vi "StateSpaceUtil_IsStabilizable.vi"(9 "B":T1, 11 "A":T1) -> (0 "Error":errorcluster, 3 "IsStabilizable":bool, 4 "Eigenvalues":cdb[](array[numeric]), 6 "R rank":i32[](array[numeric]))   [LabVIEW 2019, in "Trajectory_Library.lvlib"]
doc: "Returns true if (A, B) is a stabilizable pair.\n \n(A,B) is stabilizable if and only if the uncontrollable eigenvalues of A, if any, have absolute values less than one, where an eigenvalue is uncontrollable if rank(Lambda - A, B) < n where n is number of states.\n \nInputs:\n - A -- System matrix.\n - B -- nput matrix.\n\nOutputs:\n - IsStablizable -- If the system is stabilizable."
uses:
  Trajectory_Library.lvlib
  <vilib>/Analysis/Matrix/Datatypes/RealMatrix.ctl
  <vilib>/Analysis/Matrix/NI_Matrix.lvlib
panel:
  # "<States, States>"
  # "<States, Inputs>"
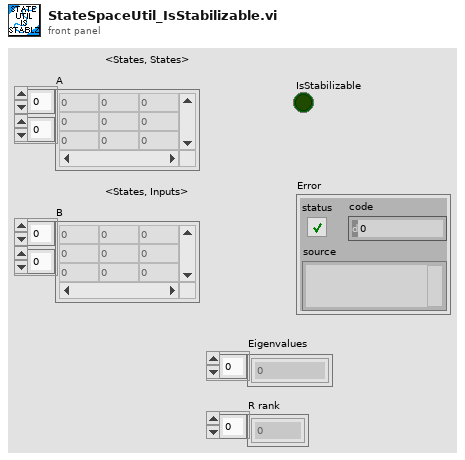
[diagram p1: front panel]
types:
  T1 = typedef "NI_Matrix.lvlib/RealMatrix.ctl" = dbl[][]
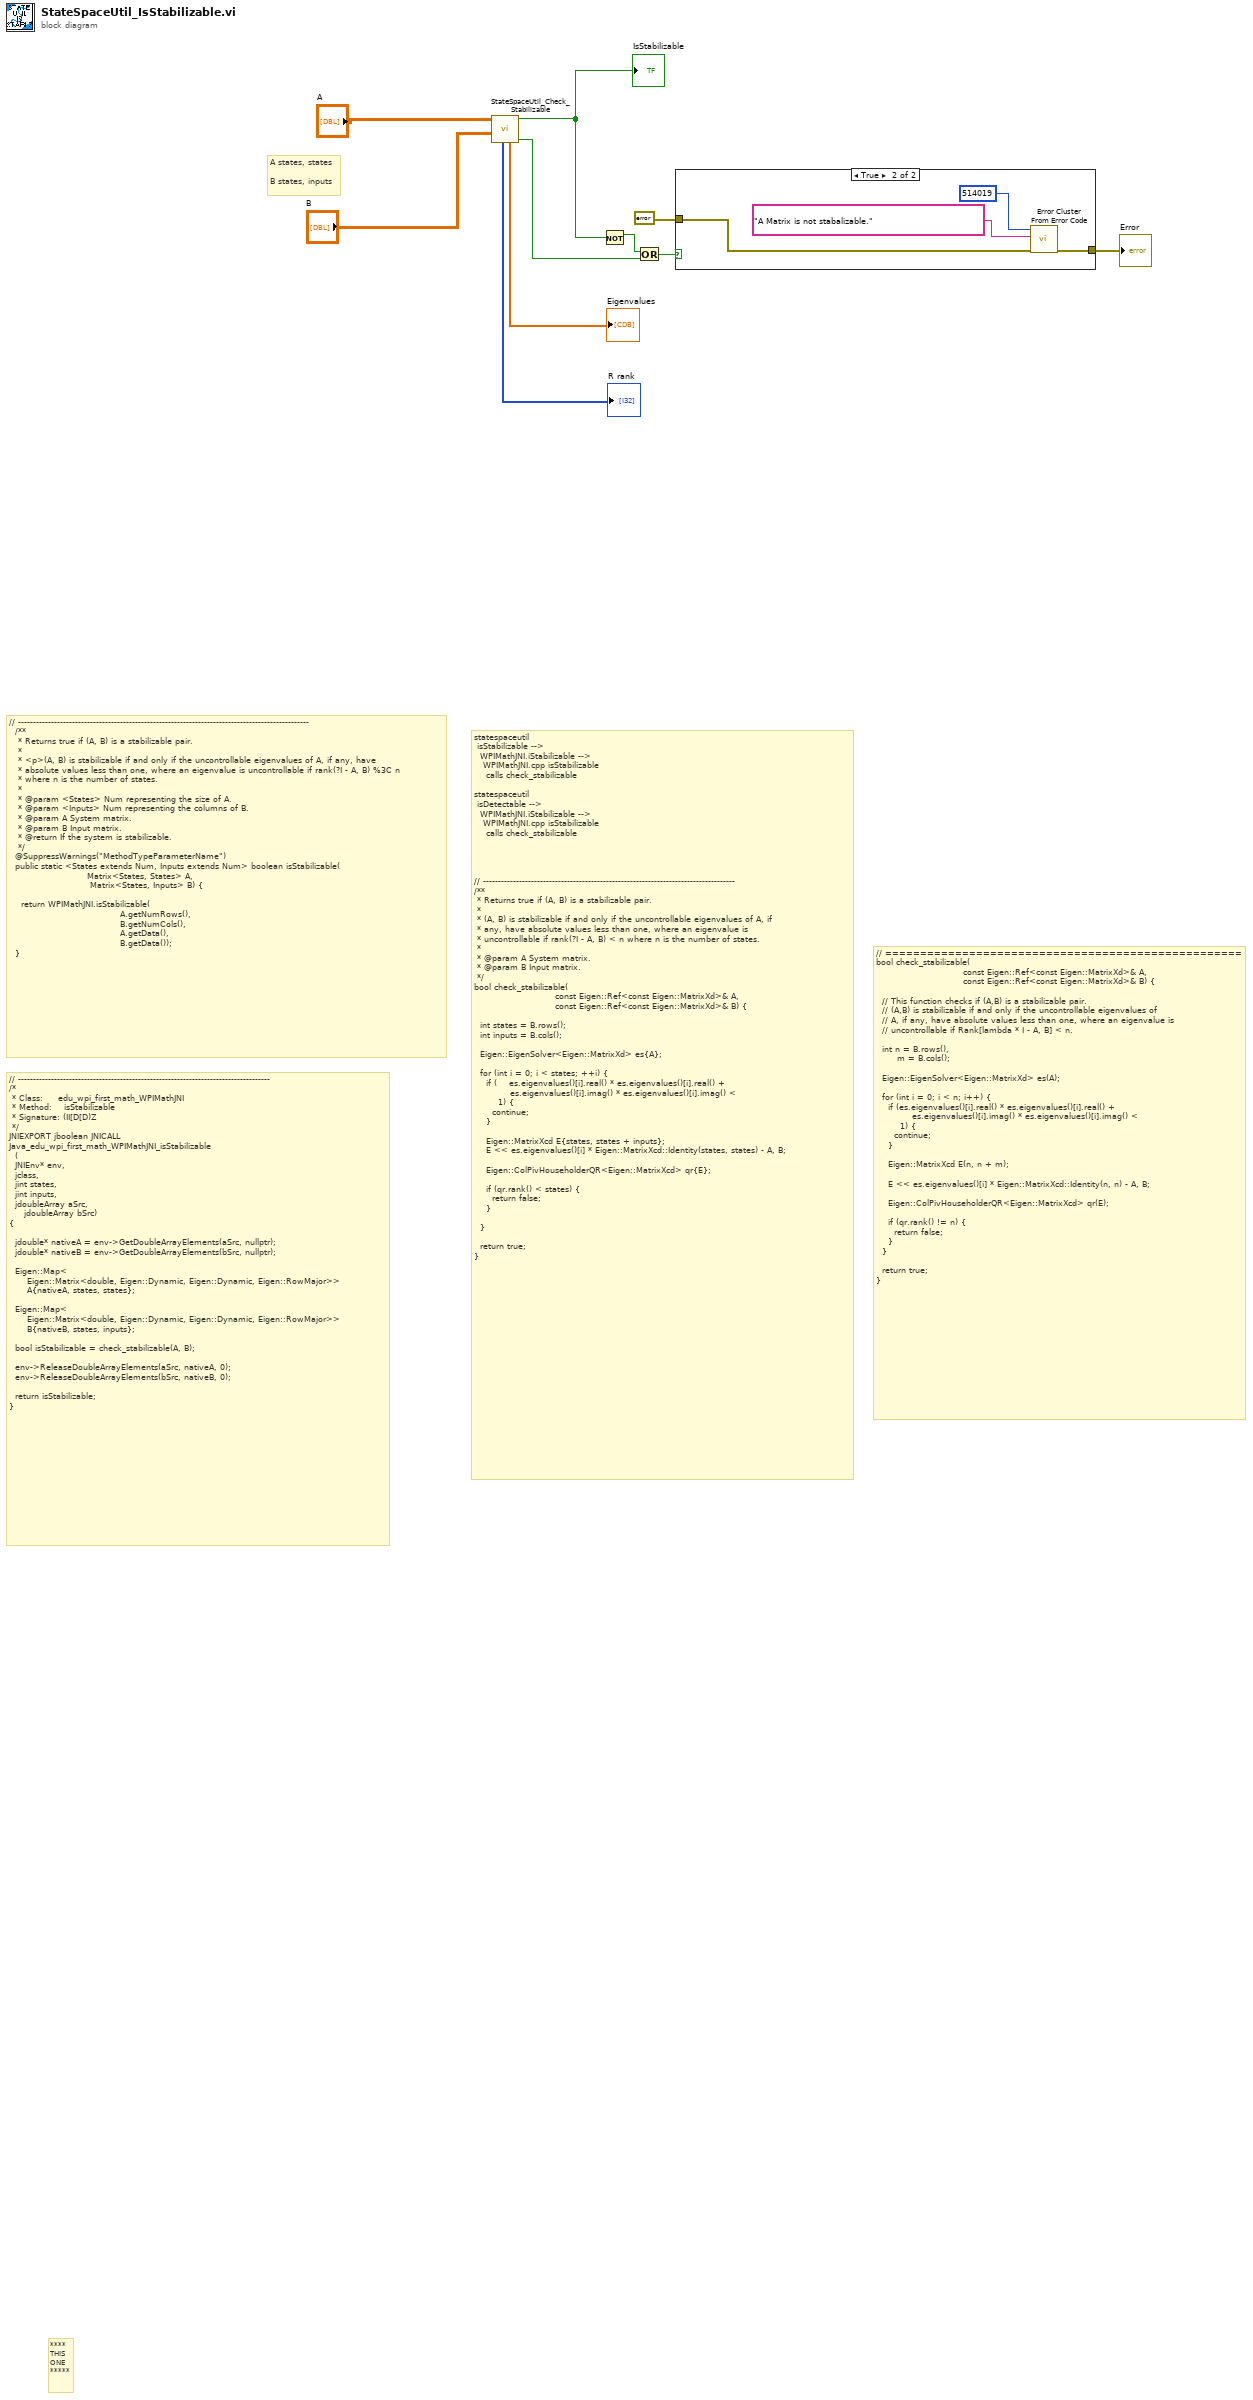
[diagram p0: block diagram]
diagram:
  # "A states, states\n\nB states, inputs"
  # "// ------------------------------------------------------------------------------------\n/*\n * Class:     edu_wpi_first_math_WPIMathJNI\n * Method:    isStabilizable\n * Signature: (II[D[D)Z\n */\nJNIEXPORT jboolean JNICALL\nJava_edu_wpi_first_math_WPIMathJNI_isStabilizable\n  (\n\t\tJNIEnv* env, \n\t\tjclass, \n\t\tjint states, \n\t\tjint inputs, \n\t\tjdoubleArray aSrc,\n   \t\tjdoubleArray bSrc)\n{\n\n  jdouble* nativeA = env->GetDoubleArrayElements(aSrc, nullptr);\n  jdouble* nativeB = env->GetDoubleArrayElements(bSrc, nullptr);\n\n  Eigen::Map<\n      Eigen::Matrix<double, Eigen::Dynamic, Eigen::Dynamic, Eigen::RowMajor>>\n      A{nativeA, states, states};\n\n  Eigen::Map<\n      Eigen::Matrix<double, Eigen::Dynamic, Eigen::Dynamic, Eigen::RowMajor>>\n      B{nativeB, states, inputs};\n\n  bool isStabilizable = check_stabilizable(A, B);\n\n  env->ReleaseDoubleArrayElements(aSrc, nativeA, 0);\n  env->ReleaseDoubleArrayElements(bSrc, nativeB, 0);\n\n  return isStabilizable;\n}"
  # "statespaceutil\n\tisStabilizable --> \n\t\tWPIMathJNI.iStabilizable --> \n\t\t\tWPIMathJNI.cpp isStabilizable  \n\t\t\t\tcalls check_stabilizable\n\nstatespaceutil\n\tisDetectable -->  \n\t\tWPIMathJNI.iStabilizable --> \n\t\t\tWPIMathJNI.cpp isStabilizable\n\t\t\t\tcalls check_stabilizable\n\n\n\n\n// ------------------------------------------------------------------------------------\n/**\n * Returns true if (A, B) is a stabilizable pair.\n *\n * (A, B) is stabilizable if and only if the uncontrollable eigenvalues of A, if\n * any, have absolute values less than one, where an eigenvalue is\n * uncontrollable if rank(?I - A, B) < n where n is the number of states.\n *\n * @param A System matrix.\n * @param B Input matrix.\n */\nbool check_stabilizable(\n                           const Eigen::Ref<const Eigen::MatrixXd>& A,\n                           const Eigen::Ref<const Eigen::MatrixXd>& B) {\n\n  int states = B.rows();\n  int inputs = B.cols();\n\n  Eigen::EigenSolver<Eigen::MatrixXd> es{A};\n\n  for (int i = 0; i < states; ++i) {\n    if (    es.eigenvalues()[i].real() * es.eigenvalues()[i].real() +\n            es.eigenvalues()[i].imag() * es.eigenvalues()[i].imag() <\n        1) {\n      continue;\n    }\n\n    Eigen::MatrixXcd E{states, states + inputs};\n    E << es.eigenvalues()[i] * Eigen::MatrixXcd::Identity(states, states) - A, B;\n\n    Eigen::ColPivHouseholderQR<Eigen::MatrixXcd> qr{E};\n\n    if (qr.rank() < states) {\n      return false;\n    }\n\n  }\n\n  return true;\n}"
  # "// ===================================================\nbool check_stabilizable(\n                             const Eigen::Ref<const Eigen::MatrixXd>& A,\n                             const Eigen::Ref<const Eigen::MatrixXd>& B) {\n\n  // This function checks if (A,B) is a stabilizable pair.\n  // (A,B) is stabilizable if and only if the uncontrollable eigenvalues of\n  // A, if any, have absolute values less than one, where an eigenvalue is\n  // uncontrollable if Rank[lambda * I - A, B] < n.\n\n  int n = B.rows(), \n       m = B.cols();\n\n  Eigen::EigenSolver<Eigen::MatrixXd> es(A);\n\n  for (int i = 0; i < n; i++) {\n    if (es.eigenvalues()[i].real() * es.eigenvalues()[i].real() +\n            es.eigenvalues()[i].imag() * es.eigenvalues()[i].imag() <\n        1) {\n      continue;\n    }\n\n    Eigen::MatrixXcd E(n, n + m);\n\n    E << es.eigenvalues()[i] * Eigen::MatrixXcd::Identity(n, n) - A, B;\n\n    Eigen::ColPivHouseholderQR<Eigen::MatrixXcd> qr(E);\n\n    if (qr.rank() != n) {\n      return false;\n    }\n  }\n\n  return true;\n}"
  # "// -------------------------------------------------------------------------------------------------\n  /**\n   * Returns true if (A, B) is a stabilizable pair.\n   *\n   * <p>(A, B) is stabilizable if and only if the uncontrollable eigenvalues of A, if any, have\n   * absolute values less than one, where an eigenvalue is uncontrollable if rank(?I - A, B) %3C n\n   * where n is the number of states.\n   *\n   * @param <States> Num representing the size of A.\n   * @param <Inputs> Num representing the columns of B.\n   * @param A System matrix.\n   * @param B Input matrix.\n   * @return If the system is stabilizable.\n   */\n  @SuppressWarnings(\"MethodTypeParameterName\")\n  public static <States extends Num, Inputs extends Num> boolean isStabilizable(\n                          Matrix<States, States> A, \n                           Matrix<States, Inputs> B) {\n\n    return WPIMathJNI.isStabilizable(\n                                   \t\tA.getNumRows(), \n                                   \t\tB.getNumCols(), \n                                   \t\tA.getData(), \n                                   \t\tB.getData());\n  }"
  # "****\nTHIS\nONE\n*****"
  n1 = call "StateSpaceUtil_Check_Stabilizable.vi"("B"="B", "A"="A") -> ("Error"=w3:bool, "IsStabilizable"=w1:bool, "Eigenvalues"=→"Eigenvalues":cdb[], "R rank"=→"R rank":i32[])  [unwired: 6 in]
  "IsStabilizable" <- w1
  n2 = Not(x=w1) -> (.not. x?=w2:bool)
  n3 = Or(x=w2, y=w3) -> (x .or. y?=w4:bool)
  n4 = case shown="True" w4 {
    tunnel: errorcluster {"status"=FALSE, "code"=0, "source"=""} ("error constant") -> [w11 w13]
    tunnel: [w11 w12] -> w5
    frame False {
    }
    frame True {
      n5 = call <vilib>:"Error Cluster From Error Code.vi"("error in (no error)"=w13, "error message (\"\")"="A Matrix is not stabalizable." ("error message (\"\")"), "error code (0)"=514019) -> ("error out"=w12:errorcluster)  [unwired: 6 in]
    }
  }
  "Error" <- w5
